vi "Read Data.vi"(8 "error in (no error)":errorcluster, 11 "DataReceived in":refnum<class "DataReceived.lvclass">) -> (0 "error out":errorcluster, 2 "Data":string, 3 "DataReceived out":refnum<class "DataReceived.lvclass">)   [LabVIEW 2022 SP3, in "TcpServer.lvlib" / "DataReceived.lvclass"]
uses:
  DataReceived.lvclass
  DataReceived.lvclass/DataReceived.ctl
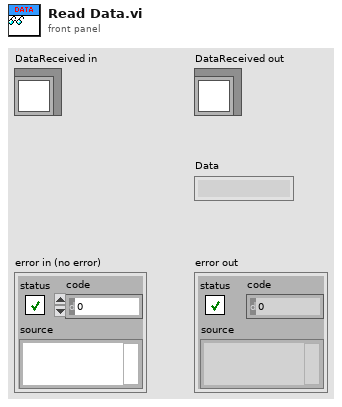
[diagram p1: front panel]
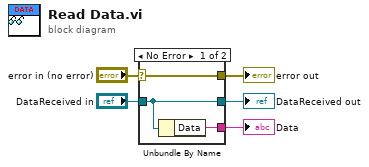
[diagram p0: block diagram]
diagram:
  n1 = case shown="No Error" "error in (no error)" {
    selector: "error in (no error)" -> [w8 w9]
    tunnel: [w8 w9] -> w4
    tunnel: [w7 w10] -> w2
    tunnel: "DataReceived in" -> [w7 w10]
    tunnel: [w6 _] -> w1
    frame No Error {
      n2 = Unbundle By Name(w7) -> ("Data"=w6:string)
    }
    frame Error {
    }
  }
  "error out" <- w4
  "DataReceived out" <- w2
  "Data" <- w1
